vi "Update plot calc.vi"(10 "Init options":T1={"UI visible?"=FALSE, "Update rate (ms)"=250, "Sidebar.Visible"=TRUE, "time to plot (init)"=600.0, "time to plot (max)"=inf, "config file start path"=path "", "Title.Visible"=TRUE, "Title"="Title", "TimeZone"=enum."Local"} {"time to plot (init)" format="%<%H:%M:%S>t"}, 11 "Loop data":T3) -> (3 "enqueue update plot?":bool)   [LabVIEW 2021, in "RocketPlot.lvlib"]
uses:
  RocketPlot.lvlib
  TypeDefs/plot while loop data.ctl
  CollapsePanel/CollapsePanel.lvclass
  TypeDefs/MouseDownState.ctl
  TypeDefs/RightClickCache.ctl
  TypeDefs/RightClickCache PlatMod.ctl
  <vilib>/Utility/miscctls.llb/LVPoint32TypeDef.ctl
  <vilib>/Utility/miscctls.llb/LVRectTypeDef.ctl
  TypeDefs/Slice average.ctl
  TypeDefs/ZoomCache.ctl
  TypeDefs/RangeCache.ctl
  <vilib>/Utility/miscctls.llb/LVRangeTypeDef.ctl
  TypeDefs/ZoomCache PlatMod.ctl
  Classes/RocketPlotHandle/SubVIs/Init Options.ctl
  TypeDefs/TimeZone.ctl
  Classes/RocketPlotHandle/RocketPlotHandle.lvclass
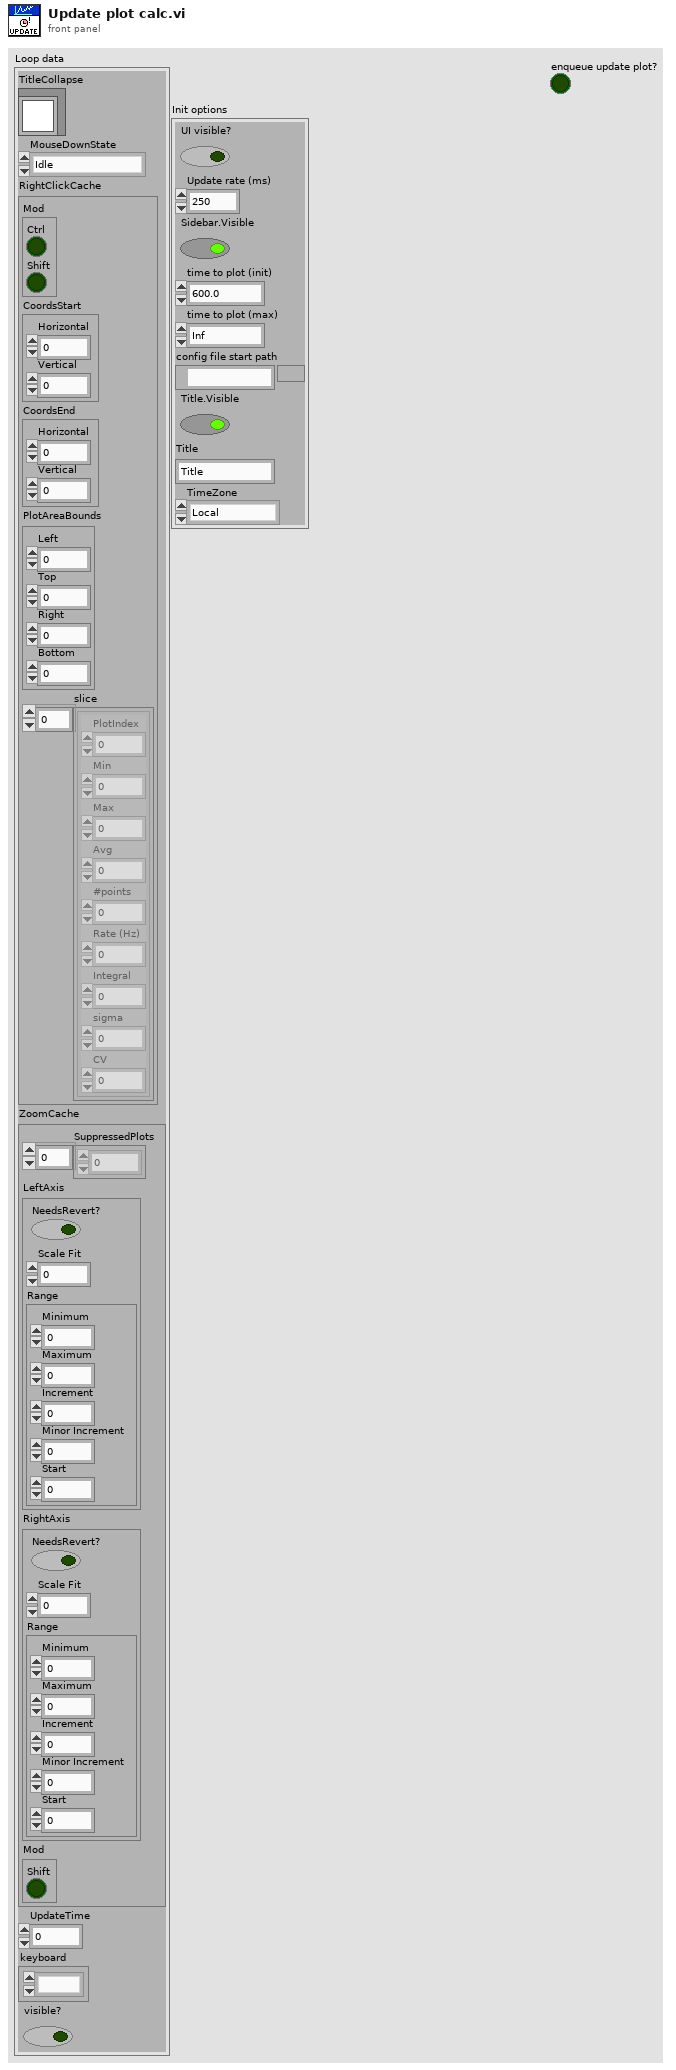
[diagram p1: front panel]
types:
  T1 = typedef "RocketPlotHandle.lvclass/Init Options.ctl" = cluster{"UI visible?":bool, "Update rate (ms)":u32, "Sidebar.Visible":bool, "time to plot (init)":dbl, "time to plot (max)":dbl, "config file start path":path, "Title.Visible":bool, "Title":string, "TimeZone":T2}
  T2 = typedef "RocketPlot.lvlib/TimeZone.ctl" = enum16{"UTC", "Local"}
  T3 = typedef "RocketPlot.lvlib/plot while loop data.ctl" = cluster{"TitleCollapse":refnum<class "CollapsePanel.lvclass">, "MouseDownState":T4, "RightClickCache":T5, "ZoomCache":T10, "UpdateTime":dbl, "keyboard":refnum<k1>, "visible?":bool}
  T4 = typedef "RocketPlot.lvlib/MouseDownState.ctl" = enum16{"Idle", "Pan", "Zoom", "Zoom-Post", "RightClick"}
  T5 = typedef "RocketPlot.lvlib/RightClickCache.ctl" = cluster{"Mod":T6, "CoordsStart":T7, "CoordsEnd":T7, "PlotAreaBounds":T8, "slice":T9[]}
  T6 = typedef "RocketPlot.lvlib/RightClickCache PlatMod.ctl" = cluster{"Ctrl":bool, "Shift":bool}
  T7 = typedef "LVPoint32TypeDef.ctl" = cluster{"Horizontal":i32, "Vertical":i32}
  T8 = typedef "LVRectTypeDef.ctl" = cluster{"Left":i16, "Top":i16, "Right":i16, "Bottom":i16}
  T9 = typedef "RocketPlot.lvlib/Slice average.ctl" = cluster{"PlotIndex":i32, "Min":dbl, "Max":dbl, "Avg":dbl, "#points":u32, "Rate (Hz)":dbl, "Integral":dbl, "sigma":dbl, "CV":dbl}
  T10 = typedef "RocketPlot.lvlib/ZoomCache.ctl" = cluster{"SuppressedPlots":i32[], "LeftAxis":T11, "RightAxis":T11, "Mod":T13}
  T11 = typedef "RocketPlot.lvlib/RangeCache.ctl" = cluster{"NeedsRevert?":bool, "Scale Fit":u8, "Range":T12}
  T12 = typedef "LVRangeTypeDef.ctl" = cluster{"Minimum":dbl, "Maximum":dbl, "Increment":dbl, "Minor Increment":dbl, "Start":dbl}
  T13 = typedef "RocketPlot.lvlib/ZoomCache PlatMod.ctl" = cluster{"Shift":bool}
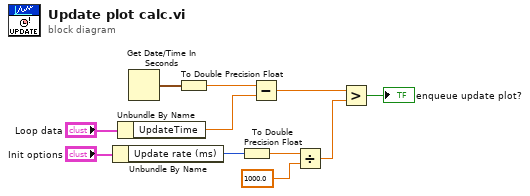
[diagram p0: block diagram]
diagram:
  n1 = Unbundle By Name("Init options") -> ("Update rate (ms)"=w7:u32)
  n2 = Unbundle By Name("Loop data") -> ("UpdateTime"=w9:dbl)
  n3 = Get Date/Time In Seconds() -> (seconds since 1Jan1904=w11:timestamp)
  n4 = To Double Precision Float(number=w11) -> (double precision float=w10:dbl)
  n5 = To Double Precision Float(number=w7) -> (double precision float=w6:dbl)
  n6 = Subtract(x=w10, y=w9) -> (x-y=w8:dbl)
  n7 = Divide(x=w6, y=1000.0) -> (x/y=w4:dbl)
  n8 = Greater?(x=w8, y=w4) -> (0:→"enqueue update plot?":bool)
